vi "OEE_SCREEN_2_display_X_axis_labels.vi"(9 "labels":string[](array[string]), 10 "labels_picture_accumulative":refnum<vi>, 11 "XYGraph in":refnum<vi>) -> ()   [LabVIEW 2019]
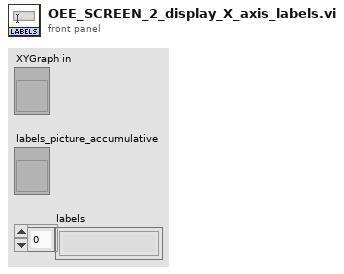
[diagram p1: front panel]
types:
  T1 = typedef "LVRectTypeDef.ctl" = cluster{"Left":i16, "Top":i16, "Right":i16, "Bottom":i16}
  T2 = cluster{"horizontal":enum16{"left", "center", "right"}, "vertical":enum16{"top", "center", "bottom"}}
  T3 = cluster{"Font Name:":string, "Size":i16, "Strikeout?":bool, "Italic?":bool, "Underline?":bool, "Outline?":bool, "Shadow?":bool, "Bold?":bool}
  T4 = enum16{"User-specified Font", "Application Font", "System Font", "Dialog Font"}
  T5 = enum16{"None", "Stacked", "Clockwise", "Counterclockwise"}
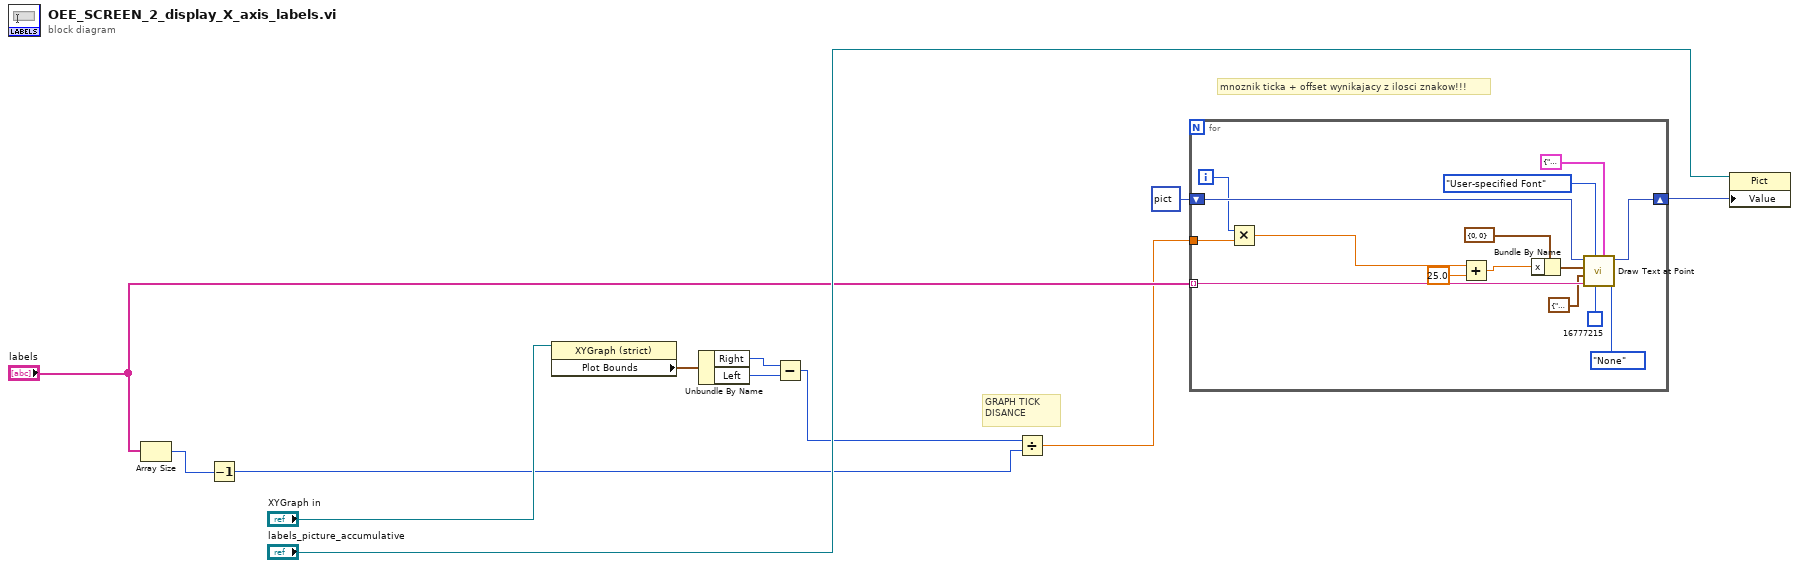
[diagram p0: block diagram]
diagram:
  # "mnoznik ticka + offset wynikajacy z ilosci znakow!!!"
  # "GRAPH TICK DISANCE"
  n1 = Array Size(array="labels") -> (size(s)=w7:i32)
  n2 = Decrement(x=w7) -> (x-1=w8:i32)
  n3 = property class="XYGraph (strict)"(reference="XYGraph in") -> ("Plot Bounds"=w10:T1)  [unwired: 1 in, 2 out]
  n4 = Unbundle By Name(w10) -> ("Right"=w6:i16, "Left"=w5:i16)
  n5 = Subtract(x=w6, y=w5) -> (x-y=w2:i16)
  n6 = Divide(x=w2, y=w8) -> (x/y=w1:dbl)
  n7 = for {
    tunnel: "labels" -> [w24] mode=indexing
    shift-right: [w26] -> w11
    shift-left: picture data[5B] ("Picture") -> [w27]
    tunnel: w1 -> [w23]
    i -> [w22]
    n8 = Multiply(x=w22, y=w23) -> (x*y=w15:dbl)
    n9 = Add(x=w15, y=25.0) -> (x+y=w13:dbl)
    n10 = Bundle By Name(cluster=cluster{"x":i16, "y":i16} {"x"=0, "y"=0} ("origin"), "x"=w13) -> (w20:cluster{"x":i16, "y":i16})
    n11 = call <vilib>:"Draw Text at Point.vi"("text orientation"=T5."None", "[user-specified font]"=T3 {"Font Name:"="Application Font", "Size"=40, "Strikeout?"=FALSE, "Italic?"=FALSE, "Underline?"=FALSE, "Outline?"=FALSE, "Shadow?"=FALSE, "Bold?"=TRUE}, "text color(black)"=u32 16777215, "desired font(Application)"=T4."User-specified Font", "text"=w24, "alignment(left, top)"=T2 {"horizontal"=enum."center", "vertical"=enum."top"}, "origin"=w20, "picture"=w27) -> ("new picture"=w26:picture)  [unwired: 2 in, 1 out]
  }
  n12 = property class="Pict"(reference="labels_picture_accumulative", "Value"=w11) -> ()  [unwired: 1 in, 2 out]
